vi "Label and Caption Color.vi"(8 "error in":errorcluster, 10 "Text Color":u32(colorbox), 11 "ctrl ref in":refnum<vi>) -> (0 "error out":errorcluster, 3 "ctrl ref out":refnum<vi>)   [LabVIEW 2021, in "TSC Material Theme.lvlib" / "Material-Scheme.lvclass"]
doc: "Color labels and captions in this subVI - running into different errors when a caption does not exist, so first I will check if the caption exists and then only color if it does so that the error shouldn't be thrown.\n\n<b>Code Developed By:</b> +\nDaniel Coons +\nTechnology Service Corporation +\nwww.tsc.com/atcs"
uses:
  Material-Scheme.lvclass
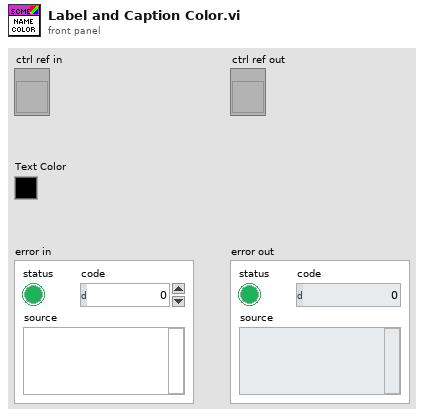
[diagram p1: front panel]
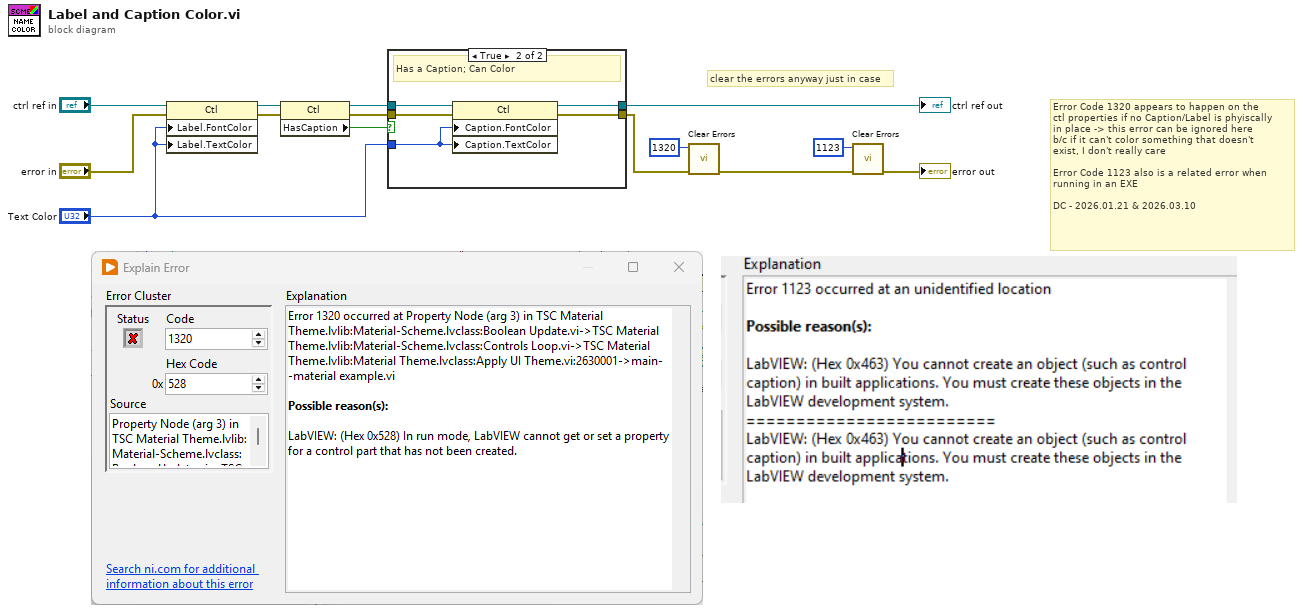
[diagram p0: block diagram]
diagram:
  # "clear the errors anyway just in case"
  # "Error Code 1320 appears to happen on the \nctl properties if no Caption/Label is phyiscally\nin place -> this error can be ignored here\nb/c if it can't color something that doesn't \nexist, I don't really care\n\nError Code 1123 also is a related error when\nrunning in an EXE\n\nDC - 2026.01.21 & 2026.03.10"
  n1 = property class="Ctl"(reference="ctrl ref in", error in="error in", "Label.FontColor"="Text Color", "Label.TextColor"="Text Color") -> (reference out=w2:refnum<vi>, error out=w9:errorcluster)
  n2 = property class="Ctl"(reference=w2, error in=w9) -> (reference out=w8:refnum<vi>, error out=w14:errorcluster, "HasCaption"=w6:bool)
  n3 = case shown="True" w6 {
    tunnel: w8 -> [w15 w19]
    tunnel: [w15 w18] -> w7
    tunnel: w14 -> [w16 w21]
    tunnel: [w16 w20] -> w13
    tunnel: "Text Color" -> [_ w17]
    frame False {
      # "no caption; so ignore to not have errors"
    }
    frame True {
      # "Has a Caption; Can Color"
      n4 = property class="Ctl"(reference=w19, error in=w21, "Caption.FontColor"=w17, "Caption.TextColor"=w17) -> (reference out=w18:refnum<vi>, error out=w20:errorcluster)
    }
  }
  "ctrl ref out" <- w7
  n5 = call <vilib>:"Clear Errors.vi"("error in (no error)"=w13, "specific error code to clear (0: all)"=1320) -> ("error out"=w11:errorcluster)  [unwired: 4 in, 1 out]
  n6 = call <vilib>:"Clear Errors.vi"("error in (no error)"=w11, "specific error code to clear (0: all)"=1123) -> ("error out"=→"error out":errorcluster)  [unwired: 4 in, 1 out]
